vi "_Set Target Object (Prot).vi"(8 "error in (no error)":errorcluster, 10 "Target Object":refnum<class "Interfaceable.lvclass">, 11 "IUnknown in":refnum<class "IUnknown.lvclass">) -> (0 "error out":errorcluster, 3 "IUnknown out":refnum<class "IUnknown.lvclass">)   [LabVIEW 2009, in "IUnknown.lvclass"]
doc: "Injects an interfaceable object into a concrete interface implementation. Concrete interfaces should use this vi when implementing interface methods. The \"target\" is the class an Interface implementation is designed for."
uses:
  IUnknown.lvclass
  Interfaceable Class/Interfaceable.lvclass
  IUnknown.lvclass/IUnknown.ctl
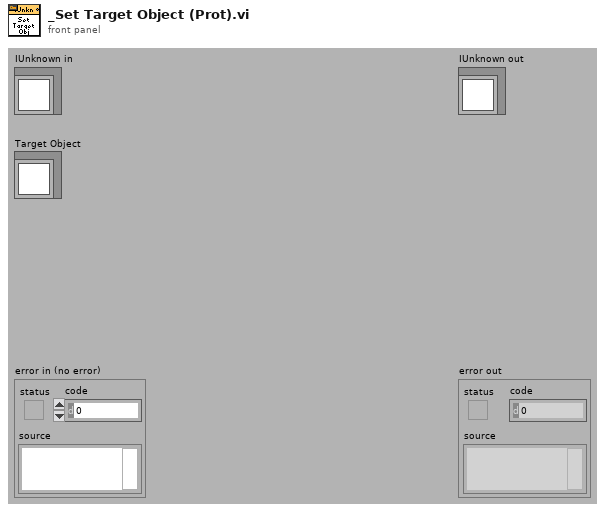
[diagram p1: front panel]
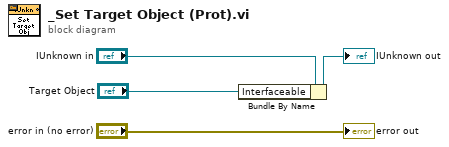
[diagram p0: block diagram]
diagram:
  n1 = Bundle By Name(cluster="IUnknown in", "Interfaceable"="Target Object") -> (→"IUnknown out":refnum<class "IUnknown.lvclass">)
  "error out" <- "error in (no error)"
